vi "create empty buffers.vi"(10 "volume info":T2) -> (2 "empty buffers":T1)   [LabVIEW 2010]
uses:
  volume_info.ctl
  projection buffers.ctl
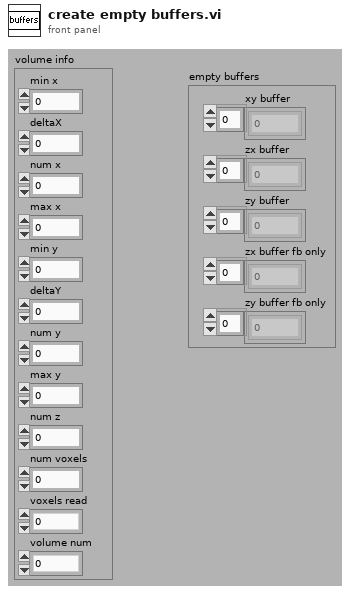
[diagram p1: front panel]
types:
  T1 = typedef "projection buffers.ctl" = cluster{"xy buffer":u32[], "zx buffer":u32[], "zy buffer":u32[], "zx buffer fb only":u32[], "zy buffer fb only":u32[]}
  T2 = typedef "volume_info.ctl" = cluster{"min x":i16, "deltaX":dbl, "num x":u32, "max x":i16, "min y":i16, "deltaY":dbl, "num y":u32, "max y":i16, "num z":u32, "num voxels":u32, "voxels read":u32, "volume num":u32}
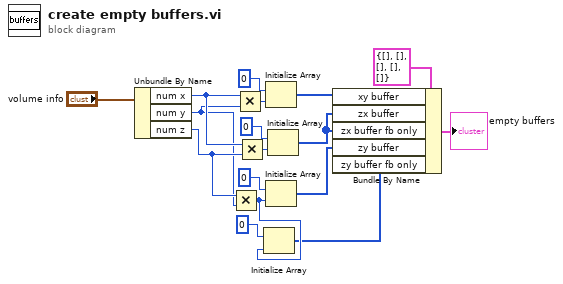
[diagram p0: block diagram]
diagram:
  n1 = Unbundle By Name("volume info") -> ("num x"=w10:u32, "num y"=w8:u32, "num z"=w9:u32)
  n2 = Multiply(x=w9, y=w8) -> (x*y=w2:u32)
  n3 = Multiply(x=w10, y=w8) -> (x*y=w15:u32)
  n4 = Multiply(x=w10, y=w9) -> (x*y=w13:u32)
  n5 = Initialize Array(u32 0, w2) -> (w1:u32[])
  n6 = Initialize Array(u32 0, w15) -> (w7:u32[])
  n7 = Initialize Array(u32 0, w2) -> (w5:u32[])
  n8 = Initialize Array(u32 0, w13) -> (w6:u32[])
  n9 = Bundle By Name(cluster=T1 {"xy buffer"=[], "zx buffer"=[], "zy buffer"=[], "zx buffer fb only"=[], "zy buffer fb only"=[]} ("buffers"), "xy buffer"=w7, "zx buffer"=w6, "zx buffer fb only"=w6, "zy buffer"=w5, "zy buffer fb only"=w1) -> (→"empty buffers":T1)
